vi "Generator Driver Template 4.vi"() -> ()   [LabVIEW 2024]
uses:
  subVIs/Revidyne Generator.lvlib
  <vilib>/addons/control/pid/NI_PID_pid.lvlib
  <vilib>/addons/control/pid/pid.llb/PID (DBL).vi
panel:
  in  "PID gains":T1={"proportional gain (Kc)"=1.0, "integral time (Ti, min)"=0.01, "derivative time (Td, min)"=0.0} {"derivative time (Td, min)" format="%.3f"; "integral time (Ti, min)" format="%.3f"; "proportional gain (Kc)" format="%.3f"}
  in  "Load":dbl(slide) scale=0.0..1000.0
  out "Waveform Chart":dbl(graph)
  in  "Speed":dbl(slide) scale=0.0..255.0
  in  "stop":bool
  in  "VISA resource name":refnum<visa-resource-name>
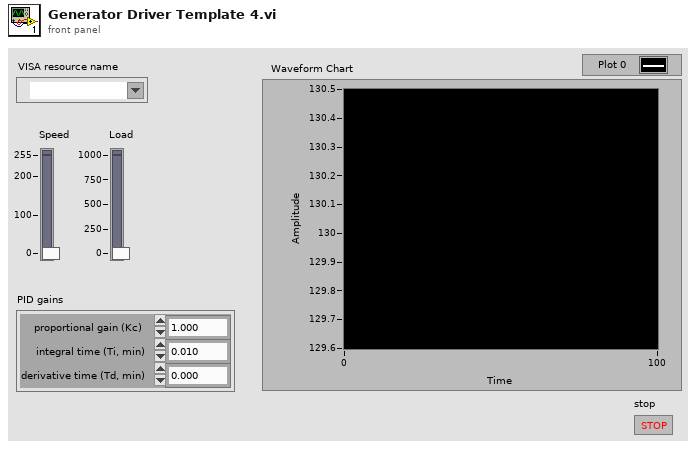
[diagram p1: front panel]
types:
  T1 = cluster{"proportional gain (Kc)":dbl, "integral time (Ti, min)":dbl, "derivative time (Td, min)":dbl}
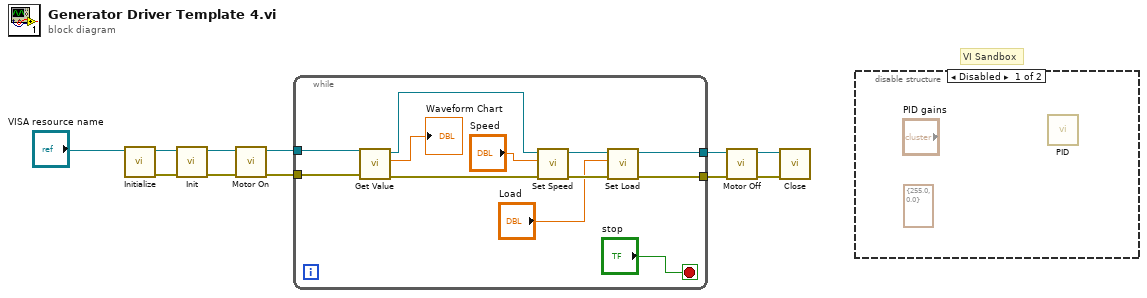
[diagram p0: block diagram]
diagram:
  # "VI Sandbox"
  n1 = call "Initialize.vi"("VISA resource name"="VISA resource name") -> ("error out"=w10:errorcluster, "VISA resource name out"=w11:refnum<visa-resource-name>)  [unwired: 9 in]
  n2 = call "Init.vi"("error in (no error)"=w10, "VISA resource name"=w11) -> ("error out"=w8:errorcluster, "VISA resource name out"=w9:refnum<visa-resource-name>)  [unwired: 8 in]
  n3 = call "Motor On.vi"("error in"=w8, "VISA resource name"=w9) -> ("error out"=w6:errorcluster, "VISA resource name out"=w7:refnum<visa-resource-name>)  [unwired: 8 in]
  n4 = while {
    tunnel: w7 -> [w23]
    tunnel: w6 -> [w22]
    tunnel: [w13] -> w4
    tunnel: [w14] -> w1
    stop <- "stop" stop-if-true
    n5 = call "Get Value.vi"("error in (no error)"=w22, "VISA resource name"=w23) -> ("error out"=w19:errorcluster, "Value"=→"Waveform Chart":dbl, "VISA resource name out"=w18:refnum<visa-resource-name>)  [unwired: 7 in]
    n6 = call "Set Speed.vi"("error in (no error)"=w19, "speed (0)"="Speed", "VISA resource name"=w18) -> ("error out"=w15:errorcluster, "VISA resource name out"=w16:refnum<visa-resource-name>)  [unwired: 7 in]
    n7 = call "Set Load.vi"("error in (no error)"=w15, "load (0)"="Load", "VISA resource name"=w16) -> ("error out"=w13:errorcluster, "VISA resource name out"=w14:refnum<visa-resource-name>)  [unwired: 7 in]
  }
  n8 = call "Motor Off.vi"("error in (no error)"=w4, "VISA resource name"=w1) -> ("error out"=w3:errorcluster, "VISA resource name out"=w5:refnum<visa-resource-name>)  [unwired: 8 in]
  n9 = call "Close.vi"("error in (no error)"=w3, "VISA resource name"=w5) -> ()  [unwired: 9 in, 1 out]
  n10 = disable-structure shown="Disabled" {
    frame Disabled {
      (unwired) cluster{"output high":dbl, "output low":dbl} {"output high"=255.0, "output low"=0.0} ("output range")
      n11 = call-poly <vilib>:"PID.vi"() -> ()  [unwired: 10 in, 2 out]
    }
    frame Enabled {
    }
  }
